vi "Execute.vi"(8 "error in (no error)":errorcluster, 9 "Consumer Queues in":T1, 10 "UI Process Command in":refnum<class "UI Display TS Panel.lvclass">, 11 "UI Process Data in":T2) -> (0 "error out":errorcluster, 1 "Consumer Queues out":T1, 2 "Stop?":bool, 3 "UI Process Data out":T2)   [LabVIEW 2019, in "User Interface Process.lvlib" / "UI Display TS Panel.lvclass"]
uses:
  UI Display TS Panel.lvclass
  UI Process Data.ctl
  TS Framework/ExeLogging/UI Logger/UI Logger.lvclass
  UI State.ctl
  TS Framework/Consumer Queues.ctl
  Generic UI Command/Generic UI Process Command.lvclass
  DAC Process/Generic DAC Command/Generic DAC Process Command.lvclass
  Trig Process/Generic Trig Command/Generic Trig Process Command.lvclass
  UI Display TS Panel.lvclass/UI Display TS Panel.ctl
  User Interface Process.lvlib
  TS Framework/TS Framework.lvlib
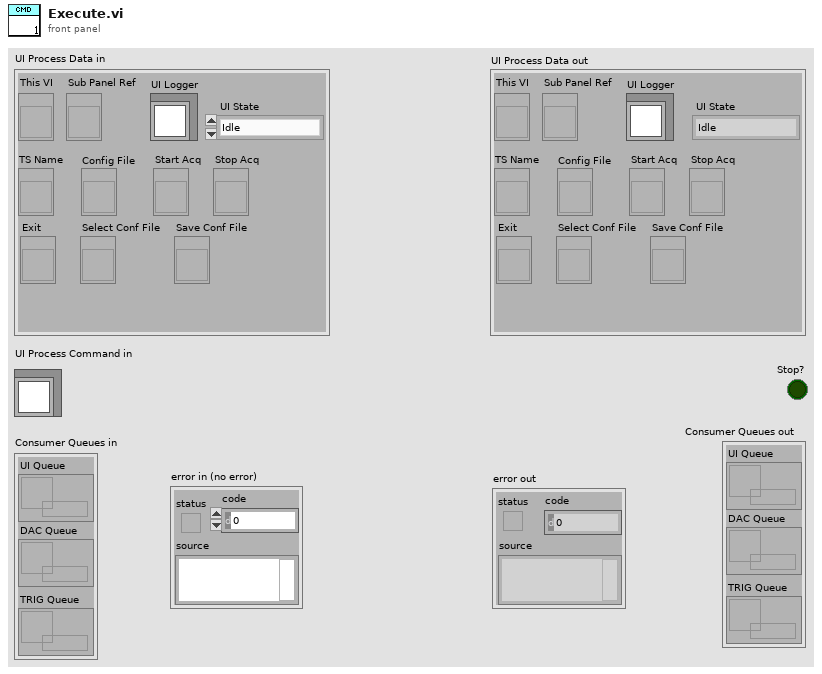
[diagram p1: front panel]
types:
  T1 = typedef "TS Framework.lvlib/Consumer Queues.ctl" = cluster{"UI Queue":refnum<queue>, "DAC Queue":refnum<queue>, "TRIG Queue":refnum<queue>}
  T2 = typedef "User Interface Process.lvlib/UI Process Data.ctl" = cluster{"This VI":refnum<vi>, "Sub Panel Ref":refnum<vi>, "UI Logger":refnum<class "UI Logger.lvclass">, "TS Name":refnum<vi>, "Config File":refnum<vi>, "Start Acq":refnum<vi>, "Stop Acq":refnum<vi>, "Exit":refnum<vi>, "Select Conf File":refnum<vi>, "Save Conf File":refnum<vi>, "UI State":T3}
  T3 = typedef "User Interface Process.lvlib/UI State.ctl" = enum16{"Idle", "Acquiring"}
  T4 = enum32{"Invalid", "Standard", "Closed", "Hidden", "Minimized", "Maximized"}
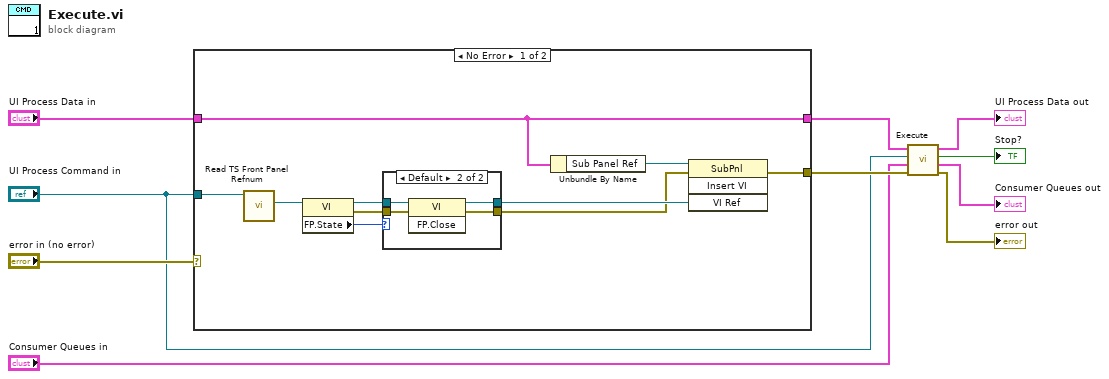
[diagram p0: block diagram]
diagram:
  n1 = case shown="No Error" "error in (no error)" {
    selector: "error in (no error)" -> [_ w27]
    tunnel: "UI Process Data in" -> [w20 w28]
    tunnel: [w20 w28] -> w4
    tunnel: [w17 w27] -> w3
    tunnel: "UI Process Command in" -> [w19 _]
    frame No Error {
      n2 = call "Read TS Front Panel Refnum.vi"("Display TS Panel in"=w19) -> ("TS Front Panel Refnum"=w12:refnum<vi>)  [unwired: 8 in, 2 out]
      n3 = property class="VI"(reference=w12) -> (reference out=w15:refnum<vi>, error out=w14:errorcluster, "FP.State"=w16:T4)  [unwired: 1 in]
      n4 = case shown="Default" w16 {
        tunnel: [w21 w26] -> w11
        tunnel: [w22 w25] -> w13
        tunnel: w15 -> [w22 w24]
        tunnel: w14 -> [w21 w23]
        frame "Closed" {
        }
        frame Default {
          n5 = invoke class="VI" method="FP.Close"(reference=w24, error in=w23) -> (reference out=w25:refnum<vi>, error out=w26:errorcluster)  [unwired: 1 in, 1 out]
        }
      }
      n6 = Unbundle By Name(w20) -> ("Sub Panel Ref"=w18:refnum<vi>)
      n7 = invoke class="SubPnl" method="Insert VI"(reference=w18, error in=w11, "VI Ref"=w13) -> (error out=w17:errorcluster)  [unwired: 1 in, 3 out]
    }
    frame Error {
    }
  }
  n8 = call-parent "Execute.vi"("error in (no error)"=w3, "Consumer Queues in"="Consumer Queues in", "UI Process Command in"="UI Process Command in", "UI Process Data in"=w4) -> ("error out"=→"error out":errorcluster, "Consumer Queues out"=→"Consumer Queues out":T1, "Stop?"=→"Stop?":bool, "UI Process Data out"=→"UI Process Data out":T2)  [unwired: 4 in]
